vi "Begin.vi"(8 "error in":errorcluster) -> (0 "error out":errorcluster)   [LabVIEW 2018]
doc: "Called before other user functions, this VI is expected to open initial I/O refnums, load in file data, and do all program initialization. Notice that the <B>error out</B> terminal is simply used for data flow. Wiring it to other structures or subVIs ensures that this VI runs first."
uses:
  <vilib>/Rock Robotics/WPI/ThirdParty/Phoenix-LabVIEW/Motor Controller/Controls/CTRE_Phoenix_MotorControl_EnhancedMotorControllerConfigurables.ctl
  <vilib>/Rock Robotics/WPI/ThirdParty/Phoenix-LabVIEW/Motor Controller/Controls/CTRE_Phoenix_MotorControl_BaseConfigurables.ctl
  <vilib>/Rock Robotics/WPI/ThirdParty/Phoenix-LabVIEW/Motor Controller/Controls/CTRE_Phoenix_MotorControl_VelocityMeasurementPeriod.ctl
  <vilib>/Rock Robotics/WPI/ThirdParty/Phoenix-LabVIEW/Motor Controller/Controls/CTRE_Phoenix_MotorControl_SlotStructure.ctl
  <vilib>/Rock Robotics/WPI/ThirdParty/Phoenix-LabVIEW/Motor Controller/Controls/CTRE_Phoenix_MotorControl_FilterStruct.ctl
  <vilib>/Rock Robotics/WPI/ThirdParty/Phoenix-LabVIEW/Motor Controller/Controls/CTRE_Phoenix_MotorControl_RemoteSourceType.ctl
  <vilib>/Rock Robotics/WPI/ThirdParty/Phoenix-LabVIEW/Controls/CTRE_Phoenix_CustomParamConfiguration.ctl
  <vilib>/Rock Robotics/WPI/ThirdParty/Phoenix-LabVIEW/Motor Controller/Controls/CTRE_Phoenix_MotorControl_FeedbackDevice.ctl
  <vilib>/Rock Robotics/WPI/ThirdParty/Phoenix-LabVIEW/Motor Controller/Controls/CTRE_Phoenix_MotorControl_SensorTermFeedbackDevice_Enhanced.ctl
  <vilib>/Rock Robotics/WPI/ThirdParty/Phoenix-LabVIEW/Motor Controller/Controls/CTRE_Phoenix_MotorControl_LimitSwitchNormal.ctl
  <vilib>/Rock Robotics/WPI/ThirdParty/Phoenix-LabVIEW/Motor Controller/Controls/CTRE_Phoenix_MotorControl_LimitSwitchSource_Local.ctl
  <vilib>/Rock Robotics/WPI/ThirdParty/Phoenix-LabVIEW/Motor Controller/Controls/CTRE_Phoenix_MotorControl_MotorControllerConfigurables.ctl
  <vilib>/Rock Robotics/WPI/ThirdParty/Phoenix-LabVIEW/Motor Controller/Controls/CTRE_Phoenix_MotorControl_RemoteFeedbackDevice.ctl
  <vilib>/Rock Robotics/WPI/ThirdParty/Phoenix-LabVIEW/Motor Controller/Controls/CTRE_Phoenix_MotorControl_SensorTermFeedbackDevice.ctl
  <vilib>/Rock Robotics/WPI/ThirdParty/Phoenix-LabVIEW/Motor Controller/Controls/CTRE_Phoenix_MotorControl_LimitSwitchSource.ctl
  <vilib>/Rock Robotics/WPI/DriverStation/WPI_DriverStationRobotMode2.ctl
  <vilib>/Rock Robotics/WPI/Joystick/WPI_JoystickDeviceEnum.ctl
  <vilib>/Rock Robotics/WPI/Solenoid/WPI_SolenoidChannel.ctl
  <vilib>/Rock Robotics/SystemInterfaces/AI/FPGA_AIChannel.ctl
  <vilib>/Rock Robotics/WPI/ThirdParty/Phoenix-LabVIEW/Motor Controller/Controls/CTRE_Phoenix_MotorControl_NeutralMode.ctl
  <vilib>/Rock Robotics/WPI/Accelerometer/WPI_AccelerometerRange.ctl
  <vilib>/Rock Robotics/WPI/ThirdParty/REV Robotics/SPARK MAX/Typedef/Spark MAX Idle Mode.ctl
  <vilib>/Rock Robotics/SystemInterfaces/DIO/FPGA_DIOPWMChannel.ctl
  Robot Global Data.vi
  RefNums_DriverStation.vi
  <vilib>/Rock Robotics/Network Tables/NT Write String Array.vi
  <vilib>/Rock Robotics/WPI/Solenoid/WPI_SolenoidOpenDouble.vi
  RefNums_Actuators.vi
  <vilib>/Rock Robotics/WPI/Utilities/WPI_GetSetVariantRefNum.vi
  RefNums_Sensors.vi
  <vilib>/Rock Robotics/WPI/Accelerometer/InternalAccelerometer/WPI_AccelerometerInternalOpen.vi
  <vilib>/Rock Robotics/WPI/Solenoid/WPI_SolenoidOpenSingle.vi
  <vilib>/Rock Robotics/WPI/SafetyOutput/WPI_SafetyOutputConfigMenu.ctl
  <vilib>/Rock Robotics/WPI/RobotDrive/WPI_RobotDriveOpen4MotorWithExistingMotors.vi
panel:
  in  "Victor Enhanced Control":T1={"Base Configurables"={"openLoopRamp"=0.0, "closedLoopRamp"=0.0, "peakOutputForward"=1.0, "peakOutputReverse"=-1.0, "nominalOutputForward"=0.0, "nominalOutputReverse"=0.0, "neutralDeadband"=0.04, "voltageCompSaturation"=0.0, "voltageMeasurementFilter"=32, "velocityMeasurementPeriod"=100, "velocityMeasurementWindow"=64, "forwardSoftLimitThreshold"=0, "reverseSoftLimitThreshold"=0, "forwardSoftLimitEnable"=FALSE, "reverseSoftLimitEnable"=FALSE, "slot0"={"P"=0.0, "I"=0.0, "D"=0.0, "F"=0.0, "integralZone"=0.0, "allowableClosedLoopError"=0, "maxIntegralAccumulator"=0.0, "closedLoopPeakOutput"=1.0, "closedLoopPeriod"=1}, "slot1"={"P"=0.0, "I"=0.0, "D"=0.0, "F"=0.0, "integralZone"=0.0, "allowableClosedLoopError"=0, "maxIntegralAccumulator"=0.0, "closedLoopPeakOutput"=1.0, "closedLoopPeriod"=1}, "slot2"={"P"=0.0, "I"=0.0, "D"=0.0, "F"=0.0, "integralZone"=0.0, "allowableClosedLoopError"=0, "maxIntegralAccumulator"=0.0, "closedLoopPeakOutput"=1.0, "closedLoopPeriod"=1}, "slot3"={"P"=0.0, "I"=0.0, "D"=0.0, "F"=0.0, "integralZone"=0.0, "allowableClosedLoopError"=0, "maxIntegralAccumulator"=0.0, "closedLoopPeakOutput"=1.0, "closedLoopPeriod"=1}, "auxPIDPolarity"=FALSE, "remoteFilter0"={"remoteSensorDeviceID"=0, "remoteSensorSource"=enum."Off"}, "remoteFilter1"={"remoteSensorDeviceID"=0, "remoteSensorSource"=enum."Off"}, "motionCruiseVelocity"=0, "motionAcceleration"=0, "motionProfileTrajectoryPeriod"=0, "feedbackNotContinuous"=FALSE, "remoteSensorClosedLoopDisableNeutralOnLOS"=FALSE, "clearPositionOnLimitF"=FALSE, "clearPositionOnLimitR"=FALSE, "clearPositionOnQuadIdx"=FALSE, "limitSwitchDisableNeutralOnLOS"=FALSE, "softLimitDisableNeutralOnLOS"=FALSE, "pulseWidthPeriod_EdgesPerRot"=1, "pulseWidthPeriod_FilterWindowSz"=1, "customParam"={"customParam0"=0, "customParam1"=0}, "trajectoryInterpolationEnable"=TRUE}, "primaryPID"={"selectedFeedbackCoefficient"=1.0, "selectedFeedbackSensor"=11}, "auxiliaryPID"={"selectedFeedbackCoefficient"=1.0, "selectedFeedbackSensor"=11}, "sum 0 term"=11, "sum 1 term"=11, "diff 0 term "=11, "diff 1 term"=11, "forwardLimitSwitchDeviceID"=0, "reverseLimitSwitchDeviceID"=0, "forwardLimitSwitchNormal"=enum."Normally Open", "reverseLimitSwitchNormal"=enum."Normally Open", "forwardLimitSwitchSource"=3, "reverseLimitSwitchSource"=3} {"diff 1 term" items=["Remote Source 0"=11, "Remote Source 1"=12, "Software Emulated"=15]; "diff 0 term" items=["Remote Source 0"=11, "Remote Source 1"=12, "Software Emulated"=15]; "sum 1 term" items=["Remote Source 0"=11, "Remote Source 1"=12, "Software Emulated"=15]; "sum 0 term" items=["Remote Source 0"=11, "Remote Source 1"=12, "Software Emulated"=15]; "reverseLimitSwitchSource" items=["Remote Talon SRX"=1, "Remote CANifier"=2, "Deactivated"=3]; "forwardLimitSwitchSource" items=["Remote Talon SRX"=1, "Remote CANifier"=2, "Deactivated"=3]; "auxiliaryPID"."selectedFeedbackSensor" items=["Sensor Sum (S0 + S1)"=9, "Sensor Difference (D0 - D1)"=10, "Remote Source 0"=11, "Remote Source 1"=12, "Software Emulated"=15]; "primaryPID"."selectedFeedbackSensor" items=["Sensor Sum (S0 + S1)"=9, "Sensor Difference (D0 - D1)"=10, "Remote Source 0"=11, "Remote Source 1"=12, "Software Emulated"=15]; "Base Configurables"."velocityMeasurementPeriod" items=["Period_1ms"=1, "Period_2ms"=2, "Period_5ms"=5, "Period_10ms"=10, "Period_20ms"=20, "Period_25ms"=25, "Period_50ms"=50, "Period_100ms"=100]}
  in  "Talon Enhanced Config":T12={"Base Configurables"={"openLoopRamp"=0.0, "closedLoopRamp"=0.0, "peakOutputForward"=1.0, "peakOutputReverse"=-1.0, "nominalOutputForward"=0.0, "nominalOutputReverse"=0.0, "neutralDeadband"=0.04, "voltageCompSaturation"=0.0, "voltageMeasurementFilter"=32, "velocityMeasurementPeriod"=100, "velocityMeasurementWindow"=64, "forwardSoftLimitThreshold"=0, "reverseSoftLimitThreshold"=0, "forwardSoftLimitEnable"=FALSE, "reverseSoftLimitEnable"=FALSE, "slot0"={"P"=0.0, "I"=0.0, "D"=0.0, "F"=0.0, "integralZone"=0.0, "allowableClosedLoopError"=0, "maxIntegralAccumulator"=0.0, "closedLoopPeakOutput"=1.0, "closedLoopPeriod"=1}, "slot1"={"P"=0.0, "I"=0.0, "D"=0.0, "F"=0.0, "integralZone"=0.0, "allowableClosedLoopError"=0, "maxIntegralAccumulator"=0.0, "closedLoopPeakOutput"=1.0, "closedLoopPeriod"=1}, "slot2"={"P"=0.0, "I"=0.0, "D"=0.0, "F"=0.0, "integralZone"=0.0, "allowableClosedLoopError"=0, "maxIntegralAccumulator"=0.0, "closedLoopPeakOutput"=1.0, "closedLoopPeriod"=1}, "slot3"={"P"=0.0, "I"=0.0, "D"=0.0, "F"=0.0, "integralZone"=0.0, "allowableClosedLoopError"=0, "maxIntegralAccumulator"=0.0, "closedLoopPeakOutput"=1.0, "closedLoopPeriod"=1}, "auxPIDPolarity"=FALSE, "remoteFilter0"={"remoteSensorDeviceID"=0, "remoteSensorSource"=enum."Off"}, "remoteFilter1"={"remoteSensorDeviceID"=0, "remoteSensorSource"=enum."Off"}, "motionCruiseVelocity"=0, "motionAcceleration"=0, "motionProfileTrajectoryPeriod"=0, "feedbackNotContinuous"=FALSE, "remoteSensorClosedLoopDisableNeutralOnLOS"=FALSE, "clearPositionOnLimitF"=FALSE, "clearPositionOnLimitR"=FALSE, "clearPositionOnQuadIdx"=FALSE, "limitSwitchDisableNeutralOnLOS"=FALSE, "softLimitDisableNeutralOnLOS"=FALSE, "pulseWidthPeriod_EdgesPerRot"=1, "pulseWidthPeriod_FilterWindowSz"=1, "customParam"={"customParam0"=0, "customParam1"=0}, "trajectoryInterpolationEnable"=TRUE}, "primaryPID"={"selectedFeedbackCoefficient"=1.0, "selectedFeedbackSensor"=0}, "auxiliaryPID"={"selectedFeedbackCoefficient"=1.0, "selectedFeedbackSensor"=0}, "sum0Term"=0, "sum1Term"=0, "diff0Term"=0, "diff1Term"=0, "forwardLimitSwitchNormal"=enum."Normally Open", "reverseLimitSwitchNormal"=enum."Normally Open", "forwardLimitSwitchDeviceID"=0, "reverseLimitSwitchDeviceID"=0, "forwardLimitSwitchSource"=enum."Feedback Connector", "reverseLimitSwitchSource"=enum."Feedback Connector", "peakCurrentLimit"=1, "peakCurrentDuration"=1, "continuousCurrentLimit"=1} {"diff1Term" items=["QuadEncoder"=0, "Analog"=2, "Tachometer"=4, "Pulse Width Encoded Position"=8, "Remote Source 0"=11, "Remote Source 1"=12, "Software Emulated"=15]; "diff0Term" items=["QuadEncoder"=0, "Analog"=2, "Tachometer"=4, "Pulse Width Encoded Position"=8, "Remote Source 0"=11, "Remote Source 1"=12, "Software Emulated"=15]; "sum1Term" items=["QuadEncoder"=0, "Analog"=2, "Tachometer"=4, "Pulse Width Encoded Position"=8, "Remote Source 0"=11, "Remote Source 1"=12, "Software Emulated"=15]; "sum0Term" items=["QuadEncoder"=0, "Analog"=2, "Tachometer"=4, "Pulse Width Encoded Position"=8, "Remote Source 0"=11, "Remote Source 1"=12, "Software Emulated"=15]; "auxiliaryPID"."selectedFeedbackSensor" items=["QuadEncoder"=0, "Analog"=2, "Tachometer"=4, "Pulse Width Encoded Position"=8, "Sensor Sum (S0 + S1)"=9, "Sensor Difference (D0 - D1)"=10, "Remote Source 0"=11, "Remote Source 1"=12, "Software Emulated"=15]; "primaryPID"."selectedFeedbackSensor" items=["QuadEncoder"=0, "Analog"=2, "Tachometer"=4, "Pulse Width Encoded Position"=8, "Sensor Sum (S0 + S1)"=9, "Sensor Difference (D0 - D1)"=10, "Remote Source 0"=11, "Remote Source 1"=12, "Software Emulated"=15]; "Base Configurables"."velocityMeasurementPeriod" items=["Period_1ms"=1, "Period_2ms"=2, "Period_5ms"=5, "Period_10ms"=10, "Period_20ms"=20, "Period_25ms"=25, "Period_50ms"=50, "Period_100ms"=100]}
  # "Sum and Diff terms are ways to select more than one sensor as a feedback device. \n Sum 0 is the first feedback device to be used for the Sum term, \n Sum 1 is the feedback device to be added to Sum 0 for the Sum term\n Diff 0 and Diff 1 work in a similar manner"
  # "These are only applicable\nif using a remote limit switch.\n\nLocal limit switches/no limit\nswitches do not use this"
  # "False: Primary Output = PID[0] + PID[1]  ---  Auxiliary Output = PID[0] - PID[1]\nTrue:  Primary Output = PID[0] - PID[1] --- Auxiliary Output = PID[0] + PID[1]"
  # "Enable the motion profile executor to perform linear interpolation between profile points.  Defaults to True."
  # "Sum and Diff terms are ways to select more than one sensor as a feedback device. \n Sum 0 is the first feedback device to be used for the Sum term.\n Sum 1 is the feedback device to be added to Sum 0 for the Sum term.\n Diff 0 and Diff 1 work in a similar manner."
  # "These are only applicable\nif using a remote limit switch.\n\nLocal limit switches/no limit\nswitches do not use this."
  # "Current is below Continuous threshold AND\n\n(Requested output is weaker** than applied motor\noutput OR is in the opposite direction).\n/\nMotor output is set to requested output."
  # "Current is above Peak* Threshold for Peak Duration.\n/\nReduce motor output (towards neutral)."
  # "Current is below Continuous threshold.\n/\nRamp motor output towards requested output."
  # "Current is above Continuous threshold.\n/\nReduce motor output (towards neutral)."
  # "Current Limiting is NOT enabled\nby default.\nCall this VI to enable."
  # "*If the configured Peak Threshold is less than the Continuous Threshold, the applied Peak Threshold is set equal to the Configured Continuous Threshold in firmware.\n** Both requested output and applied motor output are in the same direction, and requested output is closer to neutral."
  # "False: Primary Output = PID[0] + PID[1]  ---  Auxiliary Output = PID[0] - PID[1]\nTrue:  Primary Output = PID[0] - PID[1] --- Auxiliary Output = PID[0] + PID[1]"
  # "Enable the motion profile executor to perform linear interpolation between profile points.  Defaults to True."
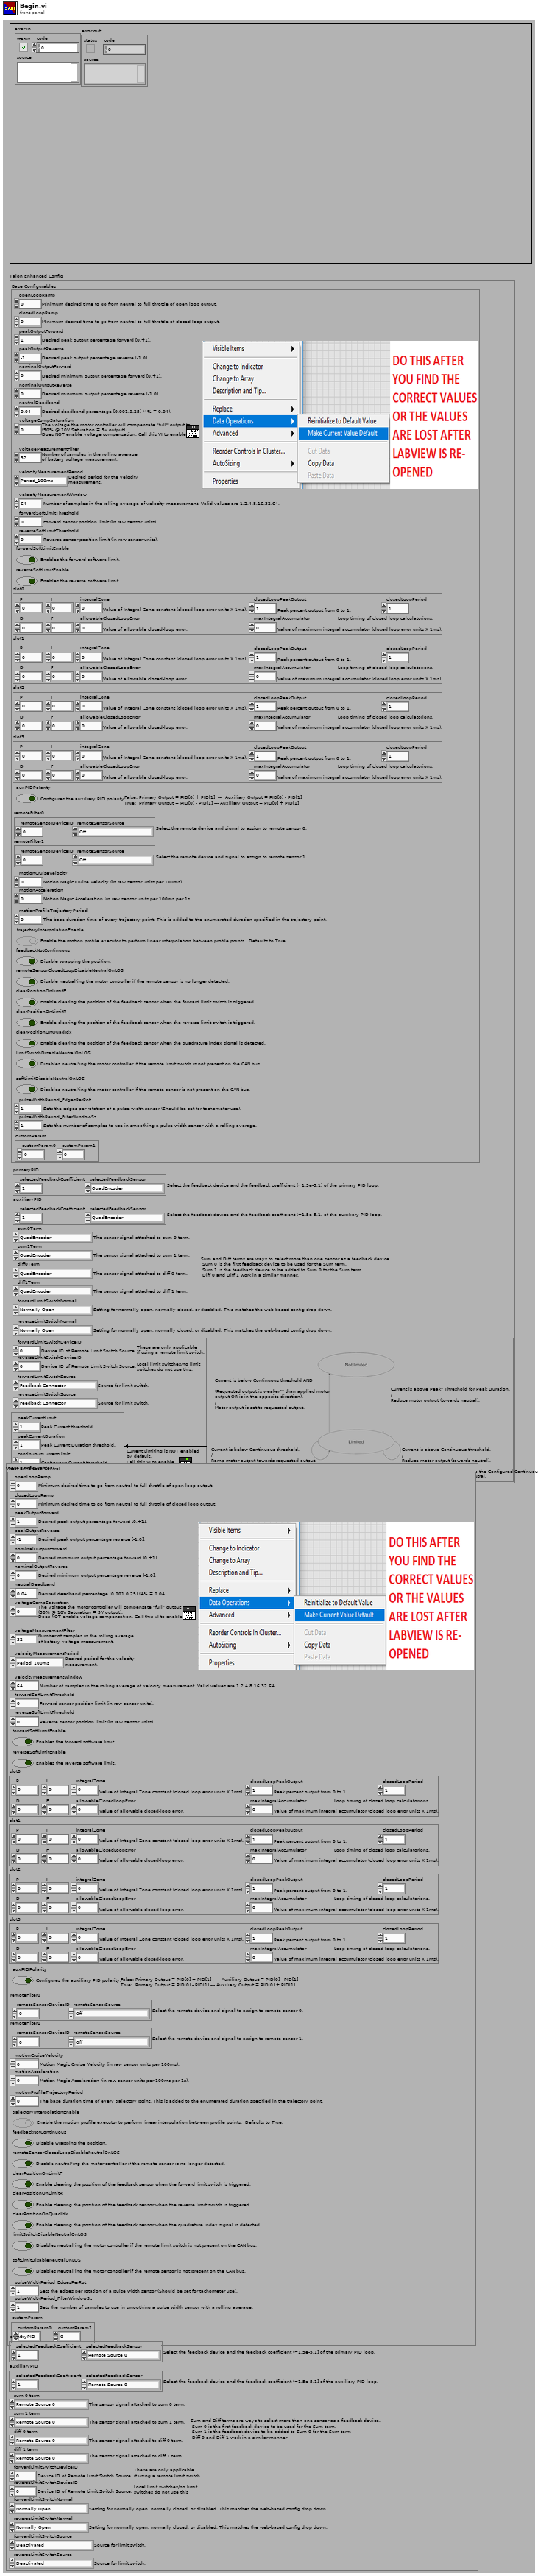
[diagram p1: front panel]
types:
  T1 = typedef "CTRE_Phoenix_MotorControl_MotorControllerConfigurables.ctl" = cluster{"Base Configurables":T2, "primaryPID":cluster{"selectedFeedbackCoefficient":dbl, "selectedFeedbackSensor":T8}, "auxiliaryPID":cluster{"selectedFeedbackCoefficient":dbl, "selectedFeedbackSensor":T8}, "sum 0 term":T9, "sum 1 term":T9, "diff 0 term ":T9, "diff 1 term":T9, "forwardLimitSwitchDeviceID":i32, "reverseLimitSwitchDeviceID":i32, "forwardLimitSwitchNormal":T10, "reverseLimitSwitchNormal":T10, "forwardLimitSwitchSource":T11, "reverseLimitSwitchSource":T11}
  T2 = typedef "CTRE_Phoenix_MotorControl_BaseConfigurables.ctl" = cluster{"openLoopRamp":dbl, "closedLoopRamp":dbl, "peakOutputForward":dbl, "peakOutputReverse":dbl, "nominalOutputForward":dbl, "nominalOutputReverse":dbl, "neutralDeadband":dbl, "voltageCompSaturation":dbl, "voltageMeasurementFilter":i32, "velocityMeasurementPeriod":T3, "velocityMeasurementWindow":i32, "forwardSoftLimitThreshold":i32, "reverseSoftLimitThreshold":i32, "forwardSoftLimitEnable":bool, "reverseSoftLimitEnable":bool, "slot0":T4, "slot1":T4, "slot2":T4, "slot3":T4, "auxPIDPolarity":bool, "remoteFilter0":T5, "remoteFilter1":T5, "motionCruiseVelocity":i32, "motionAcceleration":i32, "motionProfileTrajectoryPeriod":i32, "feedbackNotContinuous":bool, "remoteSensorClosedLoopDisableNeutralOnLOS":bool, "clearPositionOnLimitF":bool, "clearPositionOnLimitR":bool, "clearPositionOnQuadIdx":bool, "limitSwitchDisableNeutralOnLOS":bool, "softLimitDisableNeutralOnLOS":bool, "pulseWidthPeriod_EdgesPerRot":i32, "pulseWidthPeriod_FilterWindowSz":i32, "customParam":T7, "trajectoryInterpolationEnable":bool}
  T3 = typedef "CTRE_Phoenix_MotorControl_VelocityMeasurementPeriod.ctl" = u16
  T4 = typedef "CTRE_Phoenix_MotorControl_SlotStructure.ctl" = cluster{"P":dbl, "I":dbl, "D":dbl, "F":dbl, "integralZone":dbl, "allowableClosedLoopError":i32, "maxIntegralAccumulator":dbl, "closedLoopPeakOutput":dbl, "closedLoopPeriod":i32}
  T5 = typedef "CTRE_Phoenix_MotorControl_FilterStruct.ctl" = cluster{"remoteSensorDeviceID":u8, "remoteSensorSource":T6}
  T6 = typedef "CTRE_Phoenix_MotorControl_RemoteSourceType.ctl" = enum16{"Off", "Talon SRX Selected Sensor", "Pigeon IMU Yaw", "Pigeon IMU Pitch", "Pigeon IMU Roll", "CANifier Quadrature", "CANifier PWM Input 0", "CANifier PWM Input 1", "CANifier PWM Input 2", "CANifier PWM Input 3", "Gadgeteer Pigeon Yaw", "Gadgeteer Pigeon Pitch", "Gadgeteer Pigeon Roll"}
  T7 = typedef "CTRE_Phoenix_CustomParamConfiguration.ctl" = cluster{"customParam0":i32, "customParam1":i32}
  T8 = typedef "CTRE_Phoenix_MotorControl_RemoteFeedbackDevice.ctl" = i8
  T9 = typedef "CTRE_Phoenix_MotorControl_SensorTermFeedbackDevice.ctl" = i8
  T10 = typedef "CTRE_Phoenix_MotorControl_LimitSwitchNormal.ctl" = enum16{"Normally Open", "Normally Closed", "Disabled"}
  T11 = typedef "CTRE_Phoenix_MotorControl_LimitSwitchSource.ctl" = u16
  T12 = typedef "CTRE_Phoenix_MotorControl_EnhancedMotorControllerConfigurables.ctl" = cluster{"Base Configurables":T2, "primaryPID":cluster{"selectedFeedbackCoefficient":dbl, "selectedFeedbackSensor":T13}, "auxiliaryPID":cluster{"selectedFeedbackCoefficient":dbl, "selectedFeedbackSensor":T13}, "sum0Term":T14, "sum1Term":T14, "diff0Term":T14, "diff1Term":T14, "forwardLimitSwitchNormal":T10, "reverseLimitSwitchNormal":T10, "forwardLimitSwitchDeviceID":i32, "reverseLimitSwitchDeviceID":i32, "forwardLimitSwitchSource":T15, "reverseLimitSwitchSource":T15, "peakCurrentLimit":i32, "peakCurrentDuration":i32, "continuousCurrentLimit":i32}
  T13 = typedef "CTRE_Phoenix_MotorControl_FeedbackDevice.ctl" = i8
  T14 = typedef "CTRE_Phoenix_MotorControl_SensorTermFeedbackDevice_Enhanced.ctl" = i8
  T15 = typedef "CTRE_Phoenix_MotorControl_LimitSwitchSource_Local.ctl" = enum16{"Feedback Connector", "Remote Talon SRX", "Remote CANifier", "Deactivated"}
  T16 = typedef "FPGA_DIOPWMChannel.ctl" = enum8{"PWM 0", "PWM 1", "PWM 2", "PWM 3", "PWM 4", "PWM 5", "PWM 6", "PWM 7", "PWM 8", "PWM 9", "PWM MXP 0", "PWM MXP 1", "PWM MXP 2", "PWM MXP 3", "PWM MXP 4", "PWM MXP 5", "PWM MXP 6", "PWM MXP 7", "PWM MXP 8", "PWM MXP 9", "Invalid"}
  T17 = typedef "Spark MAX Idle Mode.ctl" = enum16{"Coast", "Brake"}
  T18 = typedef "WPI_SolenoidChannel.ctl" = enum8{"Solenoid 0", "Solenoid 1", "Solenoid 2", "Solenoid 3", "Solenoid 4", "Solenoid 5", "Solenoid 6", "Solenoid 7", "Invalid"}
  T19 = typedef "WPI_AccelerometerRange.ctl" = enum16{"+/- 2 g", "+/- 4 g", "+/- 8 g"}
  T20 = typedef "WPI_JoystickDeviceEnum.ctl" = enum16{"USB 0", "USB 1", "USB 2", "USB 3", "USB 4", "USB 5"}
  T21 = typedef "CTRE_Phoenix_MotorControl_NeutralMode.ctl" = enum8{"EEPROMSetting", "Override to Coast", "Override to Brake"}
  T22 = typedef "FPGA_AIChannel.ctl" = enum8{"AI 0", "AI 1", "AI 2", "AI 3", "AI MXP 0", "AI MXP 1", "AI MXP 2", "AI MXP 3", "Invalid"}
  T23 = typedef "WPI_DriverStationRobotMode2.ctl" = enum16{"Autonomous Disabled", "Autonomous Enabled", "Teleop Disabled", "Teleop Enabled", "Disconnected", "Finish", "Test Disabled", "Test Enabled", "Emergency Stopped"}
  T24 = typedef "WPI_JoystickDevRef.ctl" = cluster{"Device":T20}
  T25 = typedef "WPI_SolenoidDevRef.ctl" = cluster{"DevStatus":errorcluster, "Pneumatics Control Module":u8, "Forward Solenoid Channel":T18, "Reverse Solenoid Channel":T18}
  T26 = typedef "WPI_CompressorDevRef.ctl" = cluster{"DevStatus":errorcluster, "Pneumatics Control Module":u8}
  T27 = typedef "WPI_MotorControlDeviceRef.ctl" = cluster{"DeviceStatus":errorcluster, "Type":T28, "PWM":cluster{"PWM Channel":T16, "DeadBand":T29}, "CAN":cluster{"Device Number":u8, "SetOutput VI Ref":variant, "GetOutput VI Ref":variant, "Enable VI Ref":variant, "Disable VI Ref":variant, "Data":variant}, "Invert":bool, "DIO PWM":cluster{"PWM \"Enable\" Channel":T16, "DIOChannel":T30, "PWM Rate":dbl}}
  T28 = typedef "WPI_MotorControlType.ctl" = enum16{"PWM", "CAN", "DIO PWM"}
  T29 = typedef "WPI_PWMDeadband.ctl" = cluster{"Name":string, "maxPositivePwm":i32, "minPositivePwm":i32, "centerPwm":i32, "maxNegativePwm":i32, "minNegativePwm":i32, "angularRange":u16}
  T30 = typedef "FPGA_DIOChannel.ctl" = enum8{"DIO 0", "DIO 1", "DIO 2", "DIO 3", "DIO 4", "DIO 5", "DIO 6", "DIO 7", "DIO 8", "DIO 9", "DIO MXP 0", "DIO MXP 1", "DIO MXP 2", "DIO MXP 3", "DIO MXP 4", "DIO MXP 5", "DIO MXP 6", "DIO MXP 7", "DIO MXP 8", "DIO MXP 9", "DIO MXP 10", "DIO MXP 11", "DIO MXP 12", "DIO MXP 13", "DIO MXP 14", "DIO MXP 15", "SPI Port CS1", "SPI Port CS2", "SPI Port CS3", "SPI Port MISO", "SPI Port MOSI", "Invalid"}
  T31 = typedef "WPI_SafetyOutputConfigMenu.ctl" = enum16{"Enable", "Disable"}
  T32 = typedef "WPI_RobotDriveDevRef.ctl" = cluster{"DevStatus":errorcluster, "Motors[]":T27[], "Square Inputs":bool, "Max Output":dbl}
  T33 = typedef "WPI_ServoDeviceRef.ctl" = cluster{"DeviceStatus":errorcluster, "PWM Channel":T16, "DeadBand":T29}
  T34 = typedef "WPI_AnalogChannelDevRef.ctl" = cluster{"DevStatus":errorcluster, "Analog Channel":T22}
  T35 = typedef "WPI_AccelerometerDevRef.ctl" = cluster{"DevStatus":errorcluster, "Scaling":T36, "Analog Channels":T37, "I2C Bus":T38, "SPI Bus":T39, "Accel Range":T40, "ADXL Axes":T41, "Handle":i32, "Device Address":u8, "Accel Type":enum16{"Analog", "ADXL345 I2C", "ADXL345 SPI", "Internal", "ADXL362 SPI"}}
  T36 = typedef "WPI_AccelerometerScaling.ctl" = cluster{"Gain (VoltsPerG)":dbl, "Center Voltage":dbl}
  T37 = typedef "WPI_AccelerometerAnalogChannels.ctl" = cluster{"X-Axis":T22, "Y-Axis":T22, "Z-Axis":T22}
  T38 = typedef "i2c_bus.ctl" = enum16{"I2C On-Board", "I2C MXP", "Invalid"}
  T39 = typedef "spi_bus.ctl" = enum16{"SPI On-Board, CS0", "SPI On-Board, CS1", "SPI On-Board, CS2", "SPI On-Board, CS3", "SPI MXP", "Invalid"}
  T40 = typedef "ADXL345 Range.ctl" = u8
  T41 = typedef "WPI_AccelerometerADXL345 Axes.ctl" = cluster{"X-Axis":bool, "Y-Axis":bool, "Z-Axis":bool}
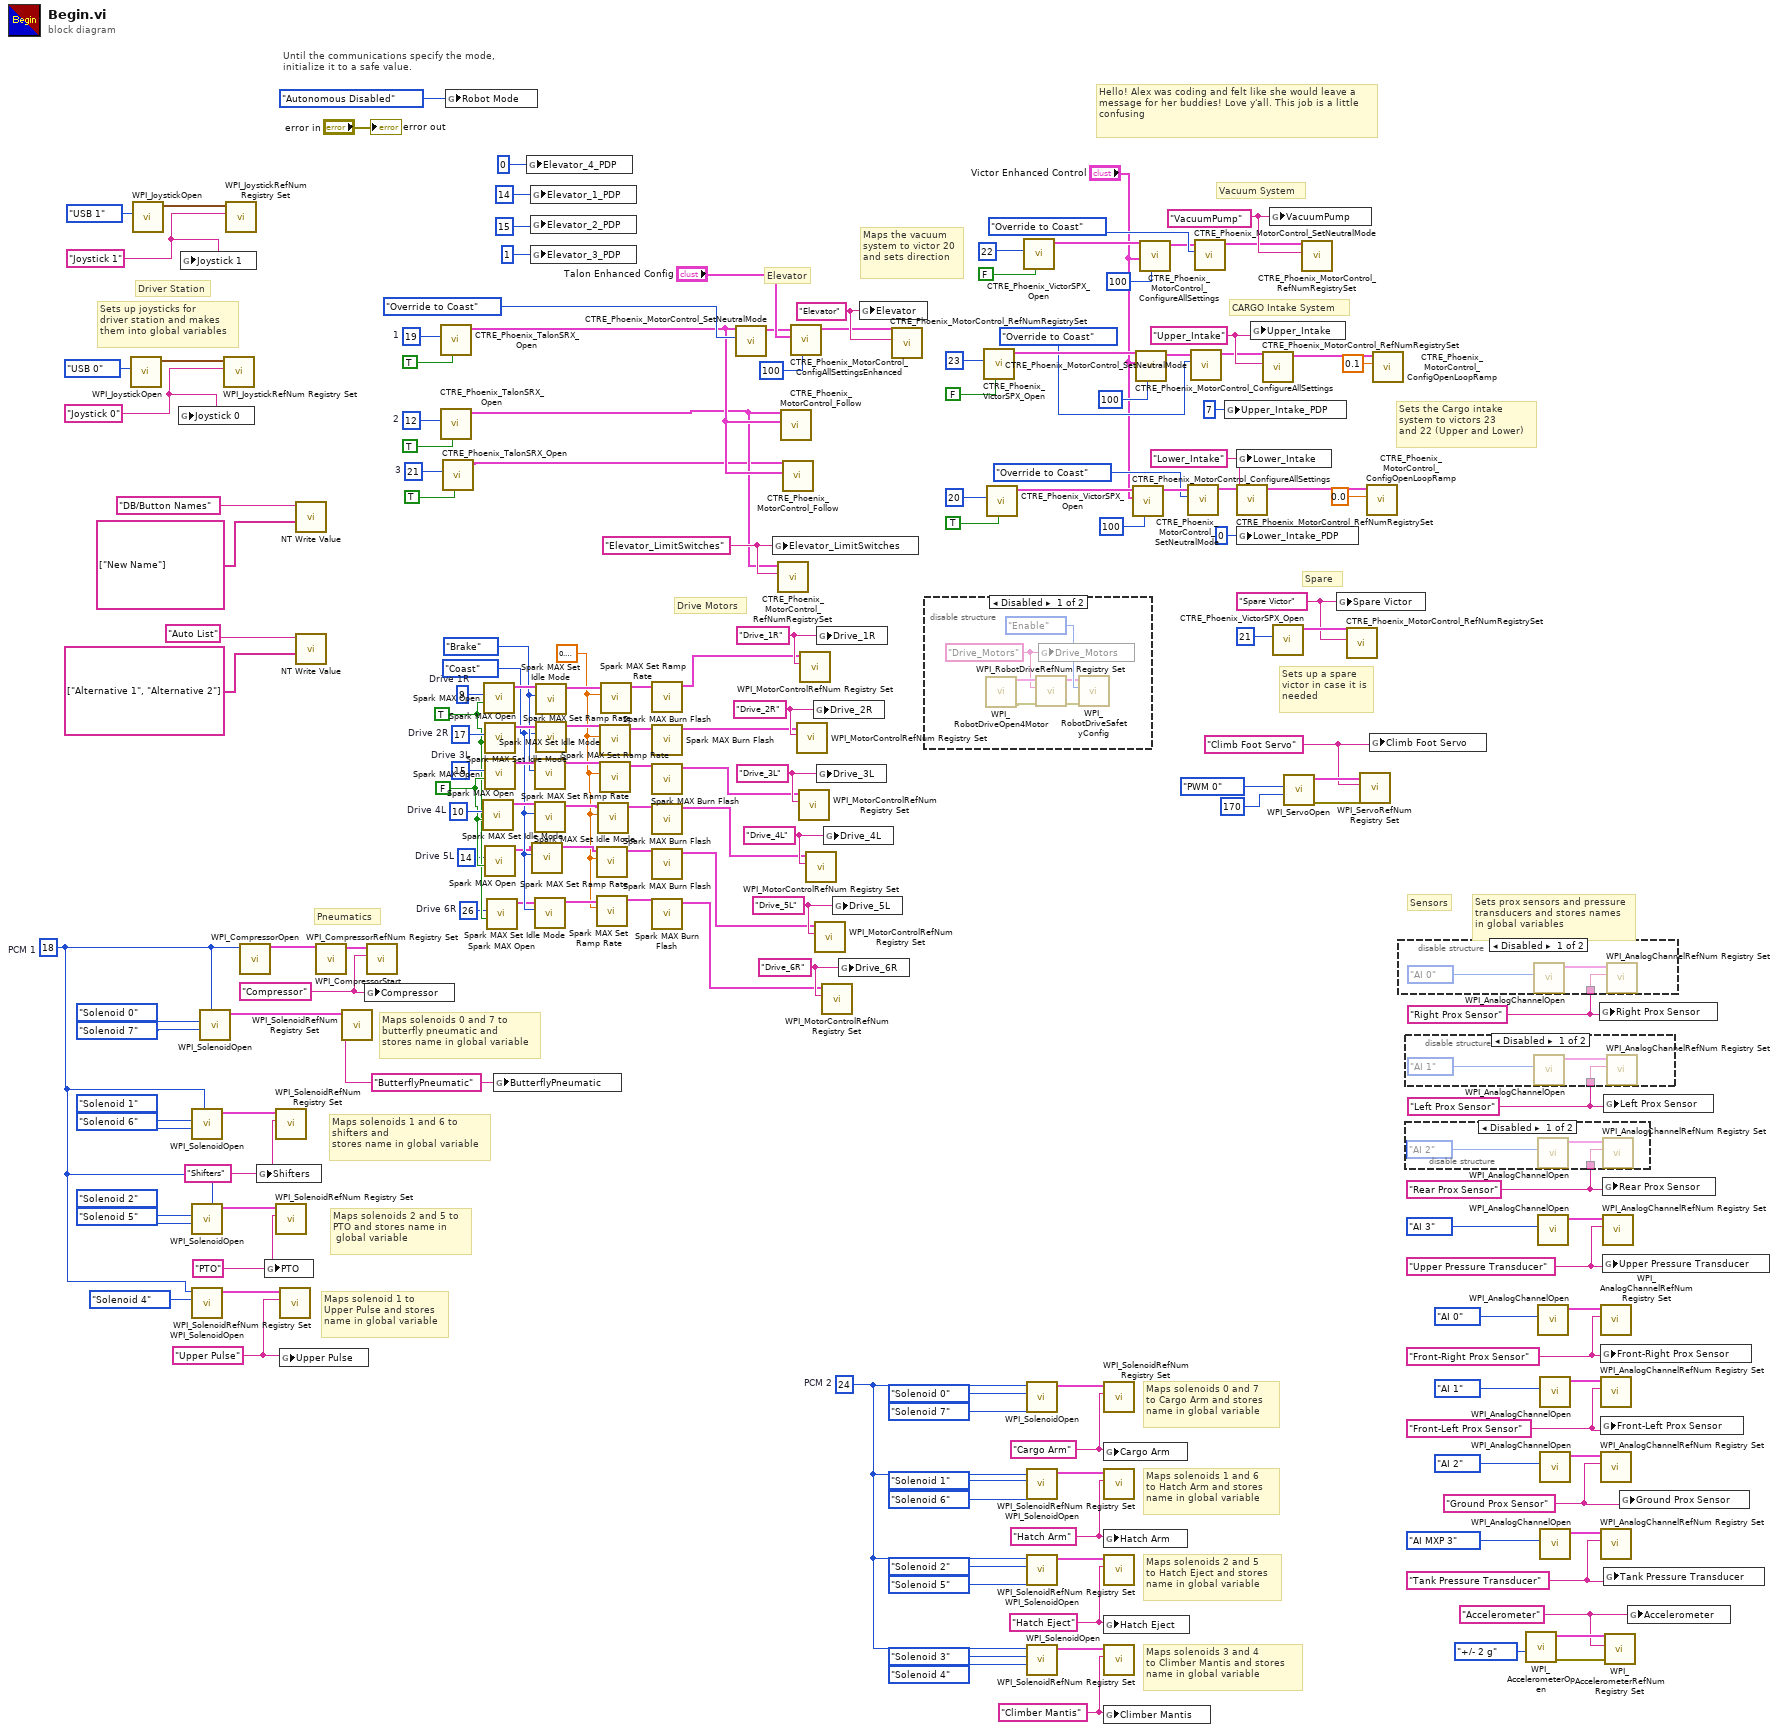
[diagram p0: block diagram]
diagram:
  w17 = u8 26  # Drive 6R
  w18 = u8 14  # Drive 5L
  w27 = "Drive_6R" ("refnum name")
  w28 = "Drive_5L" ("refnum name")
  w29 = "Climb Foot Servo" ("refnum name")
  w19 = sgl 0.1 ("Seconds from neutral to full (0)")
  w26 = Spark_MAX_Idle_Mode."Coast" ("Idle Mode")
  w46 = u8 21  # 3
  w48 = "Upper Pulse" ("ButterflyPneumatic")
  w42 = Spark_MAX_Idle_Mode."Brake" ("Idle Mode")
  w53 = "Accelerometer" ("refnum name")
  w57 = "Drive_4L" ("refnum name")
  w58 = "Drive_3L" ("refnum name")
  w59 = "Drive_2R" ("refnum name")
  w60 = "Drive_1R" ("refnum name")
  w61 = "Elevator_LimitSwitches" ("refnum name")
  w25 = FALSE ("Invert")
  w62 = u8 10  # Drive 4L
  w63 = u8 15  # Drive 3L
  w64 = u8 17  # Drive 2R
  w24 = TRUE ("Invert")
  w65 = u8 9  # Drive 1R
  w67 = "Joystick 1" ("refnum name")
  w86 = u8 12  # 2
  w91 = "Tank Pressure Transducer" ("refnum name")
  w94 = "Ground Prox Sensor" ("refnum name")
  w97 = "Front-Left Prox Sensor" ("refnum name")
  w100 = "Front-Right Prox Sensor" ("refnum name")
  w104 = "Climber Mantis" ("ButterflyPneumatic")
  w108 = "Hatch Eject" ("ButterflyPneumatic")
  w112 = "Hatch Arm" ("ButterflyPneumatic")
  w103 = u8 24  # PCM 2
  w116 = "PTO" ("ButterflyPneumatic")
  w120 = "Spare Victor" ("refnum name")
  w123 = "Upper Pressure Transducer" ("refnum name")
  w126 = "Rear Prox Sensor" ("refnum name")
  w127 = "Left Prox Sensor" ("refnum name")
  w128 = "Right Prox Sensor" ("refnum name")
  w129 = "Elevator" ("refnum name")
  w131 = u8 19  # 1
  w137 = "Lower_Intake" ("refnum name")
  w138 = "Upper_Intake" ("refnum name")
  w143 = "Cargo Arm" ("ButterflyPneumatic")
  w147 = "VacuumPump" ("refnum name")
  w150 = "Shifters" ("ButterflyPneumatic")
  w154 = "Compressor" ("Compressor")
  w155 = "ButterflyPneumatic" ("ButterflyPneumatic")
  w47 = u8 18  # PCM 1
  w161 = "Joystick 0" ("refnum name")
  # "Hello! Alex was coding and felt like she would leave a message for her buddies! Love y'all. This job is a little confusing"
  # "Maps solenoid 1 to\nUpper Pulse and stores \nname in global variable"
  # "Drive Motors"
  # "Sets the Cargo intake \nsystem to victors 23 \nand 22 (Upper and Lower)"
  # "Maps the vacuum\nsystem to victor 20\nand sets direction"
  # "Sets up a spare\nvictor in case it is\nneeded"
  # "Sets up joysticks for\ndriver station and makes\nthem into global variables"
  # "Maps solenoids 3 and 4\nto Climber Mantis and stores \nname in global variable"
  # "Maps solenoids 2 and 5\nto Hatch Eject and stores \nname in global variable"
  # "Maps solenoids 1 and 6\nto Hatch Arm and stores \nname in global variable"
  # "Maps solenoids 0 and 7\nto Cargo Arm and stores \nname in global variable"
  # "Maps solenoids 2 and 5 to\nPTO and stores name in\n global variable"
  # "Maps solenoids 1 and 6 to\nshifters and \nstores name in global variable"
  # "Maps solenoids 0 and 7 to\nbutterfly pneumatic and \nstores name in global variable"
  # "Sets prox sensors and pressure\ntransducers and stores names \nin global variables"
  # "Spare"
  # "CARGO Intake System"
  # "Vacuum System"
  # "Elevator"
  # "Sensors"
  # "Pneumatics"
  # "Driver Station"
  # "Until the communications specify the mode,\ninitialize it to a safe value."
  n1 = call <vilib>:"WPI_JoystickOpen.vi"("JoystickDevice"=WPI_JoystickDeviceEnum."USB 0") -> ("JoystickDevRef"=w168:T24)  [unwired: 10 in]
  n2 = call <vilib>:"WPI_JoystickOpen.vi"("JoystickDevice"=WPI_JoystickDeviceEnum."USB 1") -> ("JoystickDevRef"=w66:T24)  [unwired: 10 in]
  n3 = global write "RefNums_DriverStation.vi" "Joystick 0"(w161) -> ()
  n4 = global write "RefNums_DriverStation.vi" "Joystick 1"(w67) -> ()
  n5 = call-poly <vilib>:"WPI_SolenoidOpen.vi"("Reverse Solenoid Channel"=WPI_SolenoidChannel."Solenoid 6", "Forward Solenoid Channel"=WPI_SolenoidChannel."Solenoid 1", "Pneumatics Control Module (0)"=w47) -> ("SolenoidDevRef"=w151:T25)  [unwired: 7 in, 1 out]
  n6 = call-poly <vilib>:"WPI_SolenoidOpen.vi"("Reverse Solenoid Channel"=WPI_SolenoidChannel."Solenoid 5", "Forward Solenoid Channel"=WPI_SolenoidChannel."Solenoid 2", "Pneumatics Control Module (0)"=w47) -> ("SolenoidDevRef"=w117:T25)  [unwired: 7 in, 1 out]
  n7 = call-poly <vilib>:"WPI_SolenoidOpen.vi"("Solenoid Channel"=WPI_SolenoidChannel."Solenoid 4" ("Forward Solenoid Channel"), "Pneumatics Control Module (0)"=w47) -> ("SolenoidDevRef"=w49:T25)  [unwired: 8 in, 1 out]
  n8 = call-poly <vilib>:"WPI_SolenoidOpen.vi"("Reverse Solenoid Channel"=WPI_SolenoidChannel."Solenoid 7", "Forward Solenoid Channel"=WPI_SolenoidChannel."Solenoid 0", "Pneumatics Control Module (0)"=w47) -> ("SolenoidDevRef"=w157:T25)  [unwired: 7 in, 1 out]
  n9 = call <vilib>:"WPI_JoystickRefNum Registry Set.vi"("refnum name"=w161, "JoystickDevRef"=w168) -> ()  [unwired: 8 in, 2 out]
  n10 = call <vilib>:"WPI_JoystickRefNum Registry Set.vi"("refnum name"=w67, "JoystickDevRef"=w66) -> ()  [unwired: 8 in, 2 out]
  n11 = call <vilib>:"WPI_CompressorOpen.vi"("Pneumatics Control Module (0)"=w47) -> ("CompressorDevRef"=w160:T26)  [unwired: 13 in, 1 out]
  n12 = global write "RefNums_Actuators.vi" "Shifters"(w150) -> ()
  n13 = global write "RefNums_Actuators.vi" "PTO"(w116) -> ()
  n14 = call <vilib>:"WPI_SolenoidRefNum Registry Set.vi"("refnum name"=w150, "SolenoidDevRef"=w151) -> ()  [unwired: 8 in, 2 out]
  n15 = call <vilib>:"WPI_SolenoidRefNum Registry Set.vi"("refnum name"=w116, "SolenoidDevRef"=w117) -> ()  [unwired: 8 in, 2 out]
  n16 = call <vilib>:"WPI_SolenoidRefNum Registry Set.vi"("refnum name"=w48, "SolenoidDevRef"=w49) -> ()  [unwired: 8 in, 2 out]
  n17 = global write "RefNums_Actuators.vi" "Upper Pulse"(w48) -> ()
  n18 = call-poly <vilib>:"NT Write Value.vi"("String Array"=string[] ["New Name"], "Name"="DB/Button Names") -> ()  [unwired: 9 in, 1 out]
  n19 = call-poly <vilib>:"NT Write Value.vi"("String Array"=string[] ["Alternative 1", "Alternative 2"], "Name"="Auto List") -> ()  [unwired: 9 in, 1 out]
  n20 = call <vilib>:"WPI_CompressorStart.vi"("CompressorDevRef"=w160) -> ("CompressorDevRef"=w156:T26)  [unwired: 9 in, 1 out]
  n21 = call <vilib>:"WPI_SolenoidRefNum Registry Set.vi"("refnum name"=w155, "SolenoidDevRef"=w157) -> ()  [unwired: 8 in, 2 out]
  n22 = global write "RefNums_Actuators.vi" "Compressor"(w154) -> ()
  n23 = call <vilib>:"WPI_CompressorRefNum Registry Set.vi"("refnum name"=w154, "CompressorDevRef"=w156) -> ()  [unwired: 8 in, 2 out]
  n24 = call <vilib>:"CTRE_Phoenix_TalonSRX_Open.vi"("Invert"=TRUE, "Device Number"=w131) -> ("CAN Talon SRX Ref"=w15:T27)  [unwired: 8 in, 1 out]
  n25 = call <vilib>:"CTRE_Phoenix_TalonSRX_Open.vi"("Invert"=TRUE, "Device Number"=w86) -> ("CAN Talon SRX Ref"=w14:T27)  [unwired: 8 in, 1 out]
  n26 = call <vilib>:"CTRE_Phoenix_TalonSRX_Open.vi"("Invert"=TRUE, "Device Number"=w46) -> ("CAN Talon SRX Ref"=w13:T27)  [unwired: 8 in, 1 out]
  n27 = global write "Robot Global Data.vi" "Robot Mode"(WPI_DriverStationRobotMode2."Autonomous Disabled" ("Robot Mode")) -> ()
  n28 = call <vilib>:"Spark MAX Open.vi"("Invert"=w25, "Device Number"=w62) -> ("MotorControlDeviceRef"=w43:T27)  [unwired: 8 in, 1 out]
  n29 = call <vilib>:"Spark MAX Open.vi"("Invert"=w24, "Device Number"=w65) -> ("MotorControlDeviceRef"=w52:T27)  [unwired: 8 in, 1 out]
  n30 = call <vilib>:"Spark MAX Open.vi"("Invert"=w24, "Device Number"=w64) -> ("MotorControlDeviceRef"=w44:T27)  [unwired: 8 in, 1 out]
  n31 = call <vilib>:"Spark MAX Open.vi"("Invert"=w25, "Device Number"=w63) -> ("MotorControlDeviceRef"=w51:T27)  [unwired: 8 in, 1 out]
  n32 = call <vilib>:"Spark MAX Open.vi"("Invert"=w25, "Device Number"=w18) -> ("MotorControlDeviceRef"=w23:T27)  [unwired: 8 in, 1 out]
  n33 = call <vilib>:"Spark MAX Open.vi"("Invert"=w24, "Device Number"=w17) -> ("MotorControlDeviceRef"=w22:T27)  [unwired: 8 in, 1 out]
  n34 = global write "RefNums_Actuators.vi" "ButterflyPneumatic"(w155) -> ()
  n35 = global write "RefNums_Actuators.vi" "Elevator_4_PDP"(0 ("Lower_Intake_PDP")) -> ()
  n36 = global write "RefNums_Actuators.vi" "Elevator_1_PDP"(14 ("Lower_Intake_PDP")) -> ()
  n37 = global write "RefNums_Actuators.vi" "Elevator_2_PDP"(15 ("Lower_Intake_PDP")) -> ()
  n38 = global write "RefNums_Actuators.vi" "Elevator_3_PDP"(1 ("Lower_Intake_PDP")) -> ()
  n39 = call <vilib>:"Spark MAX Set Idle Mode.vi"("Idle Mode"=w26, "MotorControlDeviceRef in"=w23) -> ("MotorControlDeviceRef out"=w21:T27)  [unwired: 8 in, 1 out]
  n40 = call <vilib>:"Spark MAX Set Idle Mode.vi"("Idle Mode"=w42, "MotorControlDeviceRef in"=w51) -> ("MotorControlDeviceRef out"=w39:T27)  [unwired: 8 in, 1 out]
  n41 = call <vilib>:"Spark MAX Set Idle Mode.vi"("Idle Mode"=w26, "MotorControlDeviceRef in"=w43) -> ("MotorControlDeviceRef out"=w40:T27)  [unwired: 8 in, 1 out]
  n42 = call <vilib>:"Spark MAX Set Idle Mode.vi"("Idle Mode"=w26, "MotorControlDeviceRef in"=w22) -> ("MotorControlDeviceRef out"=w20:T27)  [unwired: 8 in, 1 out]
  n43 = call <vilib>:"Spark MAX Set Idle Mode.vi"("Idle Mode"=w42, "MotorControlDeviceRef in"=w52) -> ("MotorControlDeviceRef out"=w41:T27)  [unwired: 8 in, 1 out]
  n44 = call <vilib>:"Spark MAX Set Idle Mode.vi"("Idle Mode"=w26, "MotorControlDeviceRef in"=w44) -> ("MotorControlDeviceRef out"=w38:T27)  [unwired: 8 in, 1 out]
  n45 = call <vilib>:"Spark MAX Set Ramp Rate.vi"("Seconds from neutral to full (0)"=w19, "MotorControlDeviceRef in"=w21) -> ("MotorControlDeviceRef"=w4:T27)  [unwired: 8 in, 1 out]
  n46 = call <vilib>:"Spark MAX Set Ramp Rate.vi"("Seconds from neutral to full (0)"=w19, "MotorControlDeviceRef in"=w20) -> ("MotorControlDeviceRef"=w2:T27)  [unwired: 8 in, 1 out]
  n47 = call <vilib>:"Spark MAX Set Ramp Rate.vi"("Seconds from neutral to full (0)"=w19, "MotorControlDeviceRef in"=w40) -> ("MotorControlDeviceRef"=w6:T27)  [unwired: 8 in, 1 out]
  n48 = call <vilib>:"Spark MAX Set Ramp Rate.vi"("Seconds from neutral to full (0)"=w19, "MotorControlDeviceRef in"=w38) -> ("MotorControlDeviceRef"=w10:T27)  [unwired: 8 in, 1 out]
  n49 = call <vilib>:"Spark MAX Set Ramp Rate.vi"("Seconds from neutral to full (0)"=w19, "MotorControlDeviceRef in"=w39) -> ("MotorControlDeviceRef"=w8:T27)  [unwired: 8 in, 1 out]
  n50 = call <vilib>:"Spark MAX Set Ramp Rate.vi"("Seconds from neutral to full (0)"=w19, "MotorControlDeviceRef in"=w41) -> ("MotorControlDeviceRef"=w12:T27)  [unwired: 8 in, 1 out]
  n51 = call <vilib>:"Spark MAX Burn Flash.vi"("MotorControlDeviceRef"=w12) -> ("MotorControlDeviceRef"=w11:T27)  [unwired: 9 in, 1 out]
  n52 = call <vilib>:"Spark MAX Burn Flash.vi"("MotorControlDeviceRef"=w10) -> ("MotorControlDeviceRef"=w9:T27)  [unwired: 9 in, 1 out]
  n53 = call <vilib>:"Spark MAX Burn Flash.vi"("MotorControlDeviceRef"=w8) -> ("MotorControlDeviceRef"=w7:T27)  [unwired: 9 in, 1 out]
  n54 = call <vilib>:"Spark MAX Burn Flash.vi"("MotorControlDeviceRef"=w6) -> ("MotorControlDeviceRef"=w5:T27)  [unwired: 9 in, 1 out]
  n55 = call <vilib>:"Spark MAX Burn Flash.vi"("MotorControlDeviceRef"=w4) -> ("MotorControlDeviceRef"=w3:T27)  [unwired: 9 in, 1 out]
  n56 = call <vilib>:"Spark MAX Burn Flash.vi"("MotorControlDeviceRef"=w2) -> ("MotorControlDeviceRef"=w1:T27)  [unwired: 9 in, 1 out]
  n57 = call <vilib>:"CTRE_Phoenix_MotorControl_SetNeutralMode.vi"("Motor Control Neutral Mode"=CTRE_Phoenix_MotorControl_NeutralMode."Override to Coast", "PhoenixMotorControlDevRef"=w15) -> ("PhoenixMotorControlDevRef"=w89:T27)  [unwired: 8 in, 1 out]
  n58 = global write "RefNums_Actuators.vi" "Elevator_LimitSwitches"(w61) -> ()
  n59 = call <vilib>:"CTRE_Phoenix_MotorControl_RefNumRegistrySet.vi"("refnum name"=w61, "PhoenixMotorControlDevRef"=w14) -> ()  [unwired: 8 in, 2 out]
  n60 = call <vilib>:"CTRE_Phoenix_MotorControl_Follow.vi"("Master Controller to Follow"=w15, "PhoenixMotorControlDevRef"=w14) -> ()  [unwired: 8 in, 2 out]
  n61 = call <vilib>:"CTRE_Phoenix_MotorControl_Follow.vi"("Master Controller to Follow"=w15, "PhoenixMotorControlDevRef"=w13) -> ()  [unwired: 8 in, 2 out]
  n62 = call <vilib>:"CTRE_Phoenix_MotorControl_ConfigAllSettingsEnhanced.vi"("timeoutMs"=100, "Enhanced Motor Controller Configurables"="Talon Enhanced Config", "PhoenixMotorControlDevRef"=w89) -> ("PhoenixMotorControlDevRef"=w88:T27)  [unwired: 7 in, 1 out]
  n63 = call <vilib>:"WPI_MotorControlRefNum Registry Set.vi"("refnum name"=w59, "MotorControlDevRef"=w9) -> ()  [unwired: 8 in, 2 out]
  n64 = call <vilib>:"WPI_MotorControlRefNum Registry Set.vi"("refnum name"=w58, "MotorControlDevRef"=w7) -> ()  [unwired: 8 in, 2 out]
  n65 = call <vilib>:"WPI_MotorControlRefNum Registry Set.vi"("refnum name"=w60, "MotorControlDevRef"=w11) -> ()  [unwired: 8 in, 2 out]
  n66 = call <vilib>:"WPI_MotorControlRefNum Registry Set.vi"("refnum name"=w57, "MotorControlDevRef"=w5) -> ()  [unwired: 8 in, 2 out]
  n67 = global write "RefNums_Actuators.vi" "Drive_2R"(w59) -> ()
  n68 = call <vilib>:"WPI_MotorControlRefNum Registry Set.vi"("refnum name"=w28, "MotorControlDevRef"=w3) -> ()  [unwired: 8 in, 2 out]
  n69 = global write "RefNums_Actuators.vi" "Drive_1R"(w60) -> ()
  n70 = global write "RefNums_Actuators.vi" "Drive_3L"(w58) -> ()
  n71 = call <vilib>:"WPI_MotorControlRefNum Registry Set.vi"("refnum name"=w27, "MotorControlDevRef"=w1) -> ()  [unwired: 8 in, 2 out]
  n72 = global write "RefNums_Actuators.vi" "Drive_4L"(w57) -> ()
  n73 = global write "RefNums_Actuators.vi" "Drive_5L"(w28) -> ()
  n74 = global write "RefNums_Actuators.vi" "Drive_6R"(w27) -> ()
  n75 = global write "RefNums_Actuators.vi" "Elevator"(w129) -> ()
  n76 = call <vilib>:"CTRE_Phoenix_MotorControl_RefNumRegistrySet.vi"("refnum name"=w129, "PhoenixMotorControlDevRef"=w88) -> ()  [unwired: 8 in, 2 out]
  n77 = disable-structure shown="Disabled" {
    frame Disabled {
      w171 = "Drive_Motors" ("refnum name")
      n78 = call-poly <vilib>:"WPI_RobotDriveOpen4Motor.vi"() -> ("RobotDriveDevRef"=w173:T32, "error out"=w172:errorcluster)  [unwired: 14 in]
      n79 = call <vilib>:"WPI_RobotDriveRefNum Registry Set.vi"("error in (no error)"=w172, "refnum name"=w171, "RobotDriveDevRef"=w173) -> ("error out"=w174:errorcluster, "RobotDriveDevRef"=w175:T32)  [unwired: 7 in]
      n80 = global write "RefNums_Actuators.vi" "Drive_Motors"(w171) -> ()
      n81 = call <vilib>:"WPI_RobotDriveSafetyConfig.vi"("error in (no error)"=w174, "mode"=WPI_SafetyOutputConfigMenu."Enable", "RobotDriveDevRef"=w175) -> ()  [unwired: 7 in, 2 out]
    }
    frame Enabled {
    }
  }
  n82 = call <vilib>:"CTRE_Phoenix_VictorSPX_Open.vi"("Invert"=FALSE, "Device Number"=u8 23) -> ("CAN Talon SRX Ref"=w74:T27)  [unwired: 8 in, 1 out]
  n83 = call <vilib>:"CTRE_Phoenix_VictorSPX_Open.vi"("Invert"=TRUE, "Device Number"=u8 20) -> ("CAN Talon SRX Ref"=w73:T27)  [unwired: 8 in, 1 out]
  n84 = call <vilib>:"CTRE_Phoenix_VictorSPX_Open.vi"("Invert"=FALSE, "Device Number"=u8 22) -> ("CAN Talon SRX Ref"=w81:T27)  [unwired: 8 in, 1 out]
  n85 = call-poly <vilib>:"WPI_SolenoidOpen.vi"("Reverse Solenoid Channel"=WPI_SolenoidChannel."Solenoid 7", "Forward Solenoid Channel"=WPI_SolenoidChannel."Solenoid 0", "Pneumatics Control Module (0)"=w103) -> ("SolenoidDevRef"=w144:T25)  [unwired: 7 in, 1 out]
  n86 = call-poly <vilib>:"WPI_SolenoidOpen.vi"("Reverse Solenoid Channel"=WPI_SolenoidChannel."Solenoid 6", "Forward Solenoid Channel"=WPI_SolenoidChannel."Solenoid 1", "Pneumatics Control Module (0)"=w103) -> ("SolenoidDevRef"=w113:T25)  [unwired: 7 in, 1 out]
  n87 = call-poly <vilib>:"WPI_SolenoidOpen.vi"("Reverse Solenoid Channel"=WPI_SolenoidChannel."Solenoid 5", "Forward Solenoid Channel"=WPI_SolenoidChannel."Solenoid 2", "Pneumatics Control Module (0)"=w103) -> ("SolenoidDevRef"=w109:T25)  [unwired: 7 in, 1 out]
  n88 = call-poly <vilib>:"WPI_SolenoidOpen.vi"("Reverse Solenoid Channel"=WPI_SolenoidChannel."Solenoid 4", "Forward Solenoid Channel"=WPI_SolenoidChannel."Solenoid 3", "Pneumatics Control Module (0)"=w103) -> ("SolenoidDevRef"=w105:T25)  [unwired: 7 in, 1 out]
  n89 = call <vilib>:"WPI_SolenoidRefNum Registry Set.vi"("refnum name"=w143, "SolenoidDevRef"=w144) -> ()  [unwired: 8 in, 2 out]
  n90 = global write "RefNums_Actuators.vi" "Cargo Arm"(w143) -> ()
  n91 = call <vilib>:"WPI_SolenoidRefNum Registry Set.vi"("refnum name"=w112, "SolenoidDevRef"=w113) -> ()  [unwired: 8 in, 2 out]
  n92 = global write "RefNums_Actuators.vi" "Hatch Arm"(w112) -> ()
  n93 = call <vilib>:"WPI_SolenoidRefNum Registry Set.vi"("refnum name"=w108, "SolenoidDevRef"=w109) -> ()  [unwired: 8 in, 2 out]
  n94 = global write "RefNums_Actuators.vi" "Hatch Eject"(w108) -> ()
  n95 = call <vilib>:"WPI_SolenoidRefNum Registry Set.vi"("refnum name"=w104, "SolenoidDevRef"=w105) -> ()  [unwired: 8 in, 2 out]
  n96 = global write "RefNums_Actuators.vi" "Climber Mantis"(w104) -> ()
  n97 = call <vilib>:"CTRE_Phoenix_MotorControl_ConfigureAllSettings.vi"("timeoutMs"=100, "Motor Controller Configurables"="Victor Enhanced Control", "PhoenixMotorControlDevRef"=w73) -> ("PhoenixMotorControlDevRef"=w76:T27)  [unwired: 7 in, 1 out]
  n98 = call <vilib>:"CTRE_Phoenix_MotorControl_ConfigureAllSettings.vi"("timeoutMs"=100, "Motor Controller Configurables"="Victor Enhanced Control", "PhoenixMotorControlDevRef"=w74) -> ("PhoenixMotorControlDevRef"=w75:T27)  [unwired: 7 in, 1 out]
  n99 = call <vilib>:"CTRE_Phoenix_MotorControl_ConfigureAllSettings.vi"("timeoutMs"=100, "Motor Controller Configurables"="Victor Enhanced Control", "PhoenixMotorControlDevRef"=w81) -> ("PhoenixMotorControlDevRef"=w82:T27)  [unwired: 7 in, 1 out]
  n100 = call <vilib>:"CTRE_Phoenix_MotorControl_SetNeutralMode.vi"("Motor Control Neutral Mode"=CTRE_Phoenix_MotorControl_NeutralMode."Override to Coast", "PhoenixMotorControlDevRef"=w76) -> ("PhoenixMotorControlDevRef"=w77:T27)  [unwired: 8 in, 1 out]
  n101 = call <vilib>:"CTRE_Phoenix_MotorControl_SetNeutralMode.vi"("Motor Control Neutral Mode"=CTRE_Phoenix_MotorControl_NeutralMode."Override to Coast", "PhoenixMotorControlDevRef"=w75) -> ("PhoenixMotorControlDevRef"=w70:T27)  [unwired: 8 in, 1 out]
  n102 = call <vilib>:"CTRE_Phoenix_MotorControl_SetNeutralMode.vi"("Motor Control Neutral Mode"=CTRE_Phoenix_MotorControl_NeutralMode."Override to Coast", "PhoenixMotorControlDevRef"=w82) -> ("PhoenixMotorControlDevRef"=w84:T27)  [unwired: 8 in, 1 out]
  n103 = global write "RefNums_Actuators.vi" "Upper_Intake_PDP"(7 ("Upper_Intake_PDP")) -> ()
  n104 = global write "RefNums_Actuators.vi" "Lower_Intake"(w137) -> ()
  n105 = call <vilib>:"CTRE_Phoenix_MotorControl_RefNumRegistrySet.vi"("refnum name"=w137, "PhoenixMotorControlDevRef"=w77) -> ("PhoenixMotorControlDevRef"=w136:T27)  [unwired: 8 in, 1 out]
  n106 = global write "RefNums_Actuators.vi" "Lower_Intake_PDP"(0 ("Lower_Intake_PDP")) -> ()
  n107 = global write "RefNums_Actuators.vi" "Upper_Intake"(w138) -> ()
  n108 = call <vilib>:"CTRE_Phoenix_MotorControl_RefNumRegistrySet.vi"("refnum name"=w138, "PhoenixMotorControlDevRef"=w70) -> ("PhoenixMotorControlDevRef"=w135:T27)  [unwired: 8 in, 1 out]
  n109 = global write "RefNums_Actuators.vi" "VacuumPump"(w147) -> ()
  n110 = call <vilib>:"CTRE_Phoenix_VictorSPX_Open.vi"("Device Number"=u8 21) -> ("CAN Talon SRX Ref"=w121:T27)  [unwired: 9 in, 1 out]
  n111 = call <vilib>:"WPI_ServoOpen.vi"("Angular Range"=u16 170, "PWM Channel"=FPGA_DIOPWMChannel."PWM 0") -> ("error out"=w33:errorcluster, "ServoDeviceRef"=w30:T33)  [unwired: 8 in]
  n112 = call <vilib>:"CTRE_Phoenix_MotorControl_RefNumRegistrySet.vi"("refnum name"=w147, "PhoenixMotorControlDevRef"=w84) -> ()  [unwired: 8 in, 2 out]
  n113 = global write "RefNums_Actuators.vi" "Spare Victor"(w120) -> ()
  n114 = call <vilib>:"CTRE_Phoenix_MotorControl_RefNumRegistrySet.vi"("refnum name"=w120, "PhoenixMotorControlDevRef"=w121) -> ()  [unwired: 8 in, 2 out]
  n115 = call <vilib>:"WPI_ServoRefNum Registry Set.vi"("error in (no error)"=w33, "refnum name"=w29, "ServoDeviceRef"=w30) -> ()  [unwired: 7 in, 2 out]
  n116 = call <vilib>:"CTRE_Phoenix_MotorControl_ConfigOpenLoopRamp.vi"("secondsFromNeutralToFull"=0.0, "PhoenixMotorControlDevRef"=w136) -> ()  [unwired: 8 in, 2 out]
  n117 = global write "RefNums_Actuators.vi" "Climb Foot Servo"(w29) -> ()
  n118 = call <vilib>:"CTRE_Phoenix_MotorControl_ConfigOpenLoopRamp.vi"("secondsFromNeutralToFull"=0.1, "PhoenixMotorControlDevRef"=w135) -> ()  [unwired: 8 in, 2 out]
  n119 = disable-structure shown="Disabled" {
    disable-tunnel: w128 -> [w177 _]
    frame Disabled {
      n120 = call <vilib>:"WPI_AnalogChannelOpen.vi"("Analog Channel"=FPGA_AIChannel."AI 0") -> ("AIDeviceRef"=w179:T34)  [unwired: 9 in, 1 out]
      n121 = call <vilib>:"WPI_AnalogChannelRefNum Registry Set.vi"("refnum name"=w177, "AIDeviceRef"=w179) -> ()  [unwired: 8 in, 2 out]
    }
    frame Enabled {
    }
  }
  n122 = disable-structure shown="Disabled" {
    disable-tunnel: w127 -> [w180 _]
    frame Disabled {
      n123 = call <vilib>:"WPI_AnalogChannelOpen.vi"("Analog Channel"=FPGA_AIChannel."AI 1") -> ("AIDeviceRef"=w182:T34)  [unwired: 9 in, 1 out]
      n124 = call <vilib>:"WPI_AnalogChannelRefNum Registry Set.vi"("refnum name"=w180, "AIDeviceRef"=w182) -> ()  [unwired: 8 in, 2 out]
    }
    frame Enabled {
    }
  }
  n125 = disable-structure shown="Disabled" {
    disable-tunnel: w126 -> [w183 _]
    frame Disabled {
      n126 = call <vilib>:"WPI_AnalogChannelOpen.vi"("Analog Channel"=FPGA_AIChannel."AI 2") -> ("AIDeviceRef"=w185:T34)  [unwired: 9 in, 1 out]
      n127 = call <vilib>:"WPI_AnalogChannelRefNum Registry Set.vi"("refnum name"=w183, "AIDeviceRef"=w185) -> ()  [unwired: 8 in, 2 out]
    }
    frame Enabled {
    }
  }
  n128 = call-poly <vilib>:"WPI_AccelerometerOpen.vi"("Accel Range"=WPI_AccelerometerRange."+/- 2 g") -> ("error out"=w55:errorcluster, "AccelerometerDevRef"=w56:T35)  [unwired: 9 in]
  n129 = call <vilib>:"WPI_AnalogChannelOpen.vi"("Analog Channel"=FPGA_AIChannel."AI 3") -> ("AIDeviceRef"=w125:T34)  [unwired: 9 in, 1 out]
  n130 = call <vilib>:"WPI_AnalogChannelOpen.vi"("Analog Channel"=FPGA_AIChannel."AI 0") -> ("AIDeviceRef"=w102:T34)  [unwired: 9 in, 1 out]
  n131 = call <vilib>:"WPI_AnalogChannelOpen.vi"("Analog Channel"=FPGA_AIChannel."AI 1") -> ("AIDeviceRef"=w99:T34)  [unwired: 9 in, 1 out]
  n132 = call <vilib>:"WPI_AnalogChannelOpen.vi"("Analog Channel"=FPGA_AIChannel."AI 2") -> ("AIDeviceRef"=w96:T34)  [unwired: 9 in, 1 out]
  n133 = call <vilib>:"WPI_AnalogChannelOpen.vi"("Analog Channel"=FPGA_AIChannel."AI MXP 3") -> ("AIDeviceRef"=w93:T34)  [unwired: 9 in, 1 out]
  n134 = global write "RefNums_Sensors.vi" "Right Prox Sensor"(w128) -> ()
  n135 = call <vilib>:"WPI_AnalogChannelRefNum Registry Set.vi"("refnum name"=w100, "AIDeviceRef"=w102) -> ()  [unwired: 8 in, 2 out]
  n136 = global write "RefNums_Sensors.vi" "Front-Right Prox Sensor"(w100) -> ()
  n137 = call <vilib>:"WPI_AnalogChannelRefNum Registry Set.vi"("refnum name"=w97, "AIDeviceRef"=w99) -> ()  [unwired: 8 in, 2 out]
  n138 = global write "RefNums_Sensors.vi" "Front-Left Prox Sensor"(w97) -> ()
  n139 = call <vilib>:"WPI_AnalogChannelRefNum Registry Set.vi"("refnum name"=w94, "AIDeviceRef"=w96) -> ()  [unwired: 8 in, 2 out]
  n140 = call <vilib>:"WPI_AnalogChannelRefNum Registry Set.vi"("refnum name"=w91, "AIDeviceRef"=w93) -> ()  [unwired: 8 in, 2 out]
  n141 = global write "RefNums_Sensors.vi" "Rear Prox Sensor"(w126) -> ()
  n142 = call <vilib>:"WPI_AnalogChannelRefNum Registry Set.vi"("refnum name"=w123, "AIDeviceRef"=w125) -> ()  [unwired: 8 in, 2 out]
  n143 = global write "RefNums_Sensors.vi" "Upper Pressure Transducer"(w123) -> ()
  n144 = global write "RefNums_Sensors.vi" "Left Prox Sensor"(w127) -> ()
  n145 = global write "RefNums_Sensors.vi" "Tank Pressure Transducer"(w91) -> ()
  n146 = call <vilib>:"WPI_AccelerometerRefNum Registry Set.vi"("error in (no error)"=w55, "refnum name"=w53, "AccelerometerDevRef"=w56) -> ()  [unwired: 7 in, 2 out]
  n147 = global write "RefNums_Sensors.vi" "Ground Prox Sensor"(w94) -> ()
  n148 = global write "RefNums_Sensors.vi" "Accelerometer"(w53) -> ()
  "error out" <- "error in"
